vi "GetTh.vi"(0 "class data in":refnum<class "AnalogComparator.lvclass">) -> (6 "configAnalogComp.Threshold":dbl)   [LabVIEW 2019, in "AnalogComparator.lvclass"]
uses:
  AnalogComparator.lvclass
  AnalogComparator.lvclass/AnalogComparator.ctl
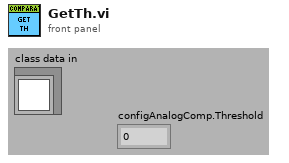
[diagram p1: front panel]
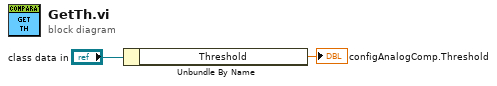
[diagram p0: block diagram]
diagram:
  n1 = Unbundle By Name("class data in") -> ("Threshold"=→"configAnalogComp.Threshold":dbl)
